vi "SyringeZCalibration.vi"(4 "AssmbType":enum16{"Sensor", "HB"}(ring), 5 "ModuleName":string="T1", 6 "Position":enum16{"1", "2"}(ring), 7 "Zone":enum16{"ZoneA", "ZoneB", "ZoneC", "ZoneD"}(ring), 8 "Error In":errorcluster, 9 "SyringeToPlateGap(mm)":dbl=0.35, 10 "PD_Z":bool=TRUE, 11 "AutoFocus":bool=TRUE) -> (0 "error out":errorcluster, 1 "HighVSPosition":picture, 2 "Image":T2(plugin-control), 3 "FinalZ":dbl)   [LabVIEW 2019]
uses:
  <vilib>/Utility/file.llb/Read Delimited Spreadsheet (DBL).vi
  include/GlobalVariables.vi
panel:
  out "CurrentZvalue":dbl
  out "AF_Zs":string
  out "SyringeZwriteTo":string
  out "OffsetUsed":dbl
  in  "Offset = -(AF_Z + PD_Z - FinalZ_needed - Gap)":T1={"BP_Zoffset(Si_assembly)"=-68.2905, "Sensor_Zoffset(HB_assembly)"=-68.3505}
  out "AF_MinZ":dbl
  out "AF_OutputPlotFile":string
  out "AF_OutputTextFile":string
  out "AF_InputTextFile":string
  out "VatPD_Z":dbl
  out "MeasuredPD_Z":dbl
  out "Vmid":dbl
  out "Vmin":dbl
  out "Vstart":dbl
  out "Vmax":dbl
  # "MainInputs"
  # "MainOutputs"
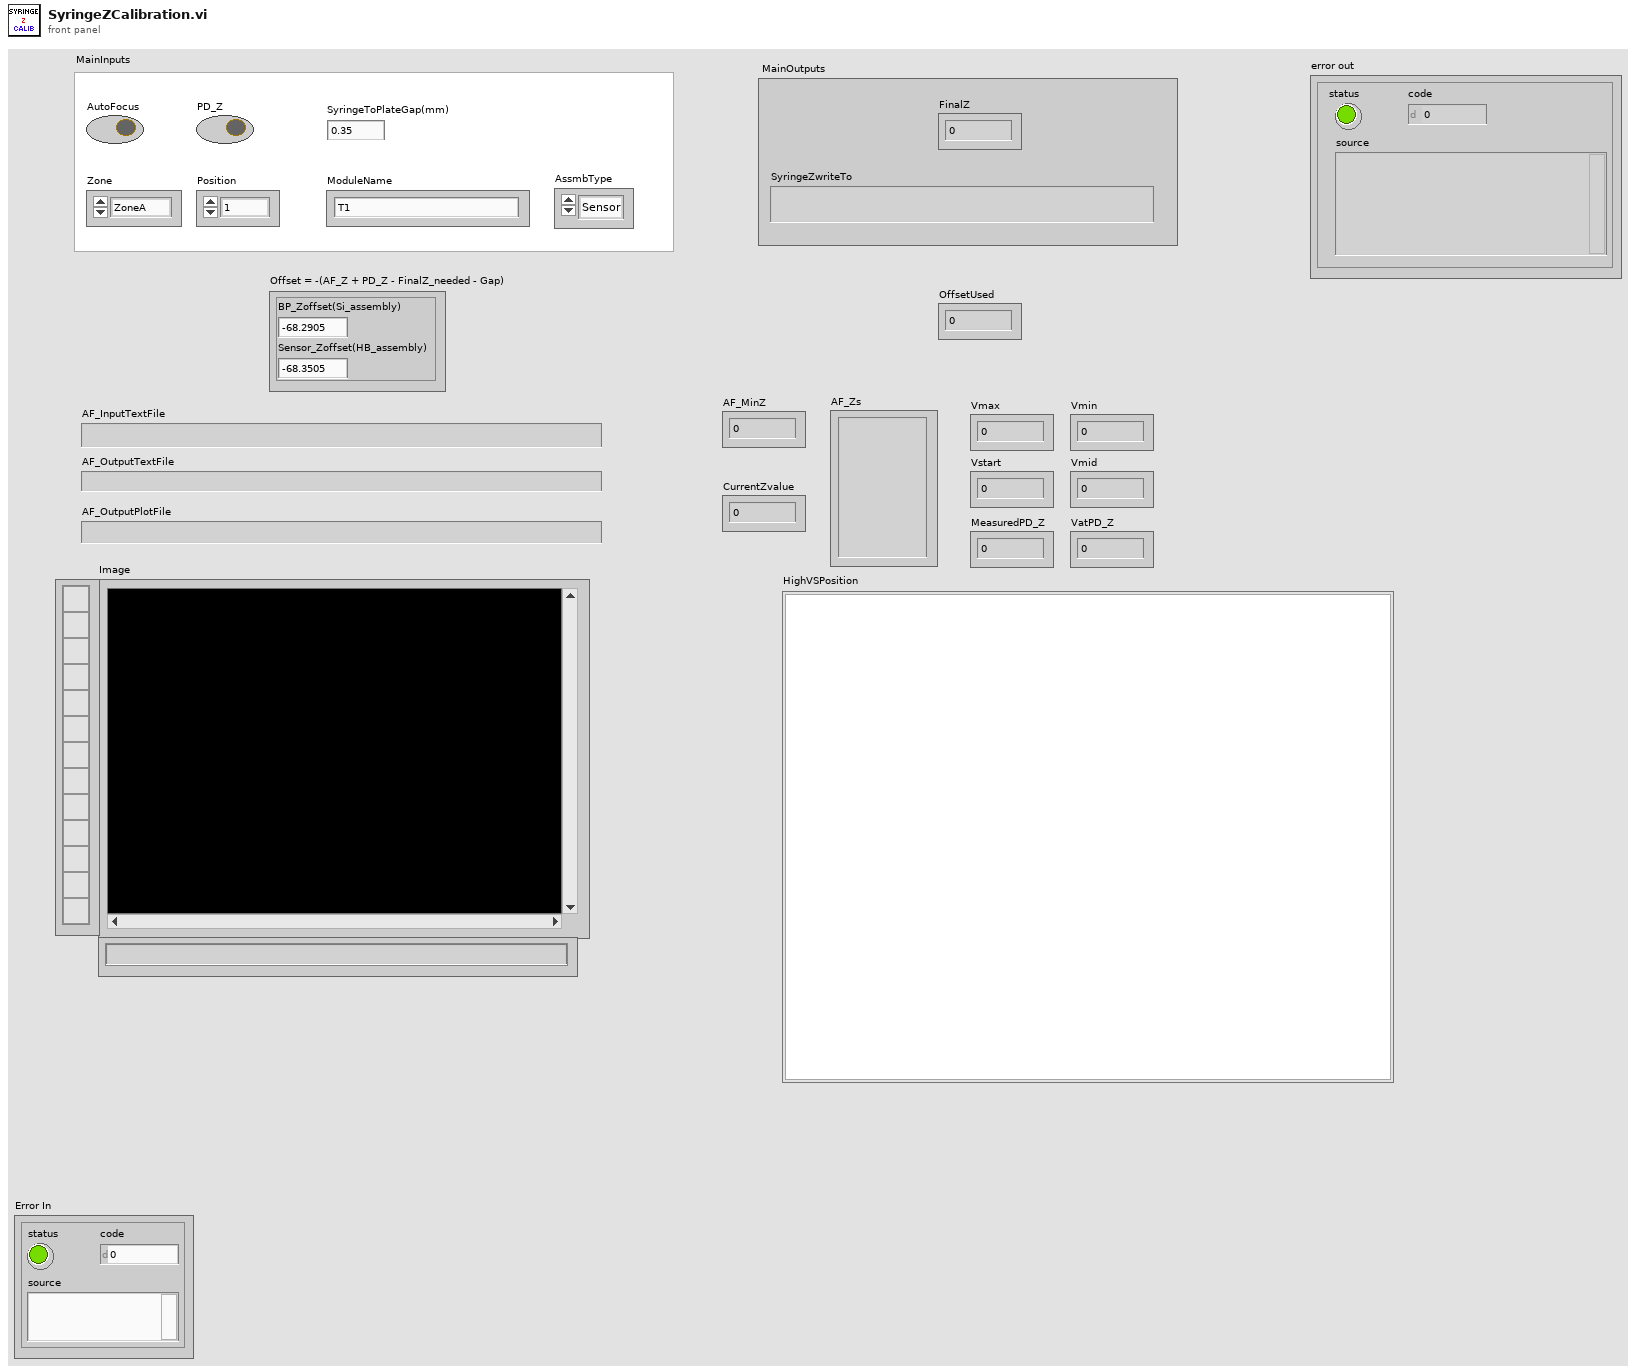
[diagram p1: front panel]
types:
  T1 = cluster{"BP_Zoffset(Si_assembly)":dbl, "Sensor_Zoffset(HB_assembly)":dbl}
  T2 = typedef "IMAQ Image.ctl" = refnum<image>
  T3 = enum16{"open", "replace", "create", "open or create", "replace or create", "replace or create with confirmation"}
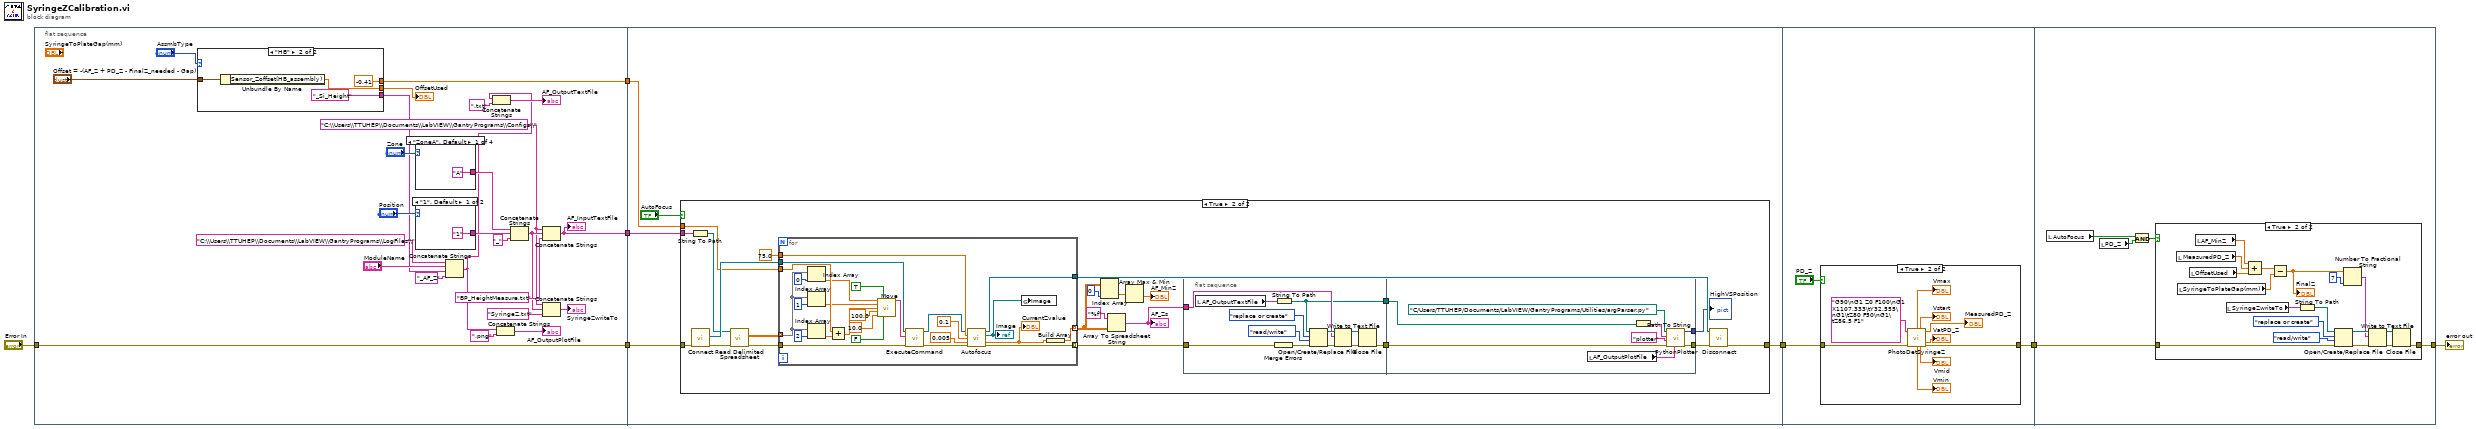
[diagram p0: block diagram]
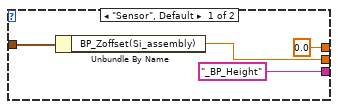
[diagram p2: hidden frame]
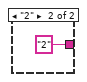
[diagram p3: hidden frame]
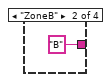
[diagram p4: hidden frame]
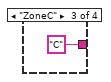
[diagram p5: hidden frame]
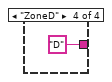
[diagram p6: hidden frame]
diagram:
  n1 = flat-sequence {
    tunnel: "Error In" -> [w20]
    tunnel: [w20] -> w5
    tunnel: [w27] -> w4
    tunnel: [w25] -> w3
    tunnel: w5 -> [w51]
    tunnel: w4 -> [w48]
    tunnel: w3 -> [w47]
    tunnel: [w49] -> w2
    tunnel: w2 -> [w122]
    tunnel: [w121] -> w1
    tunnel: [w134] -> w7
    tunnel: w1 -> [w135]
    frame #0 {
      w12 = "C:\\Users\\TTUHEP\\Documents\\LabVIEW\\GantryPrograms\\Configs\\"
      n2 = case shown="\"HB\"" "AssmbType" {
        tunnel: [0.0 -0.41] -> w27
        tunnel: "Offset = -(AF_Z + PD_Z - FinalZ_needed - Gap)" -> [w35 w39]
        tunnel: [w34 w38] -> w9
        tunnel: ["_BP_Height" "_Si_Height"] -> w8
        frame "Sensor", Default {
          n3 = Unbundle By Name(w35) -> ("BP_Zoffset(Si_assembly)"=w34:dbl)
        }
        frame "HB" {
          n4 = Unbundle By Name(w39) -> ("Sensor_Zoffset(HB_assembly)"=w38:dbl)
        }
      }
      "OffsetUsed" <- w9
      n5 = case shown="\"ZoneA\", Default" "Zone" {
        tunnel: ["A" "B" "C" "D"] -> w31
        frame "ZoneA", Default {
        }
        frame "ZoneB" {
        }
        frame "ZoneC" {
        }
        frame "ZoneD" {
        }
      }
      n6 = case shown="\"1\", Default" "Position" {
        tunnel: ["1" "2"] -> w32
        frame "1", Default {
        }
        frame "2" {
        }
      }
      n7 = Concatenate Strings("C:\\Users\\TTUHEP\\Documents\\LabVIEW\\GantryPrograms\\LogFiles\\", "ModuleName", w8, "_AF_Z" ("string")) -> (w16:string)
      n8 = Concatenate Strings(w16, ".txt" ("string")) -> (→"AF_OutputTextFile":string)
      n9 = Concatenate Strings(w16, ".png" ("string")) -> (→"AF_OutputPlotFile":string)
      n10 = Concatenate Strings(w31, w32, "_" ("string")) -> (w14:string)
      n11 = Concatenate Strings(w12, w14, "BP_HeightMeasure.txt" ("string")) -> (w25:string)
      "AF_InputTextFile" <- w25
      n12 = Concatenate Strings(w12, w14, "SyringeZ.txt" ("string")) -> (→"SyringeZwriteTo":string)
    }
    frame #1 {
      n13 = case shown="True" "AutoFocus" {
        tunnel: w51 -> [w52 w61]
        tunnel: [w52 w60] -> w49
        tunnel: w48 -> [_ w59]
        tunnel: w47 -> [_ w57]
        frame False {
        }
        frame True {
          n14 = String To Path(string=w57) -> (path=w58:path)
          n15 = call "Connect.vi"("error in (no error)"=w61) -> ("error out"=w71:errorcluster, "controller"=w72:refnum<k24>)  [unwired: 9 in]
          n16 = call-poly <vilib>:"Read Delimited Spreadsheet.vi"("file path (dialog if empty)"=w58, "error in (no error)"=w71) -> ("all rows"=w67:dbl[][], "error out"=w63:errorcluster)  [unwired: 8 in, 4 out]
          n17 = for {
            tunnel: w67 -> [w117] mode=indexing
            tunnel: w63 -> [w99]
            tunnel: [w115] -> w66 mode=indexing
            tunnel: [w114] -> w55 mode=indexing
            tunnel: w72 -> [w101]
            tunnel: [w113] -> w69
            tunnel: 75.0 ("SafeMaxZ") -> [w110]
            tunnel: w59 -> [w112]
            n18 = Index Array(array=w117, index=0) -> (element=w109:dbl)
            n19 = Index Array(array=w117, index=1) -> (element=w108:dbl)
            n20 = Index Array(array=w117, index=2) -> (element=w111:dbl)
            n21 = Add(x=w112, y=w111) -> (x+y=w107:dbl)
            n22 = call "Move.vi"("X"=w109, "Absolute"=TRUE, "Y"=w108, "Z"=w107, "SpeedXY (mm/s)"=100.0, "SpeedZ (mm/s)"=10.0, "Move Z first"=FALSE) -> ("Position Gcode"=w102:string)  [unwired: 8 in]
            n23 = call "ExecuteCommand.vi"("error in (no error)"=w99, "Command Code"=w102, "controller in"=w101) -> ("error out"=w98:errorcluster, "controller out"=w100:refnum<k24>)  [unwired: 6 in, 1 out]
            n24 = call "Autofocus.vi"("controller in"=w100, "SafeMaxZ"=w110, "InitialStepSize"=0.1, "Tolerance"=0.005, "error in (no error)"=w98) -> ("controller out"=w113:refnum<k24>, "Image"=w95:T2, "BestZvalue"=w116:dbl, "error out"=w115:errorcluster)  [unwired: 6 in, 1 out]
            "Image" <- w95
            "CurrentZvalue" <- w116
            n25 = global write "GlobalVariables.vi" "Image"(w95) -> ()
            n26 = Build Array(w116) -> (w114:dbl[])
          }
          n27 = Index Array(array=w55, index (col)=0 ("disabled index (col)")) -> (element=w53:dbl[])  [unwired: 1 in]
          n28 = Array To Spreadsheet String(array=w55, 3:"%f" ("format string")) -> (spreadsheet string=w64:string)  [unwired: 1 in]
          "AF_Zs" <- w64
          n29 = Array Max & Min(array=w53) -> (min value=→"AF_MinZ":dbl)  [unwired: 3 out]
          n30 = flat-sequence {
            tunnel: w66 -> [w86]
            tunnel: w64 -> [w79]
            tunnel: [w77] -> w74
            tunnel: [w76] -> w73
            tunnel: w74 -> [w94]
            tunnel: [w93] -> w70
            tunnel: [w92] -> w62
            tunnel: w73 -> [w89]
            frame #0 {
              n31 = local read "AF_OutputTextFile"() -> (w75:string)
              n32 = Merge Errors(w86) -> (w78:errorcluster)
              n33 = String To Path(string=w75) -> (path=w76:path)
              n34 = Open/Create/Replace File(file path (use dialog)=w76, error in=w78, operation (0:open)=T3."replace or create", access (0:read/write)=enum16{"read/write", "read-only", "write-only"}."read/write") -> (refnum out=w82:refnum<file>, error out=w83:errorcluster)  [unwired: 2 in, 1 out]
              n35 = Write to Text File(file (use dialog)=w82, text=w79, error in=w83) -> (refnum out=w85:refnum<file>, error out=w84:errorcluster)  [unwired: 1 in, 1 out]
              n36 = Close File(refnum=w85, error in=w84) -> (error out=w77:errorcluster)  [unwired: 1 out]
            }
            frame #1 {
              n37 = local read "AF_OutputPlotFile"() -> (w87:string)
              n38 = Path To String(path=w89) -> (string=w90:string)
              n39 = call "PythonPlotter.vi"("Output File"=w87, "error in (no error)"=w94, "Function Name"="plotter", "Input File"=w90, "Python Path"=path "C:/Users/TTUHEP/Documents/LabVIEW/GantryPrograms/Utilities/argParser.py") -> ("error out"=w93:errorcluster, "HighVSPosition"=w92:picture)  [unwired: 4 in]
            }
          }
          n40 = call "Disconnect.vi"("error in (no error)"=w70, "controller"=w69) -> ("error out"=w60:errorcluster)  [unwired: 9 in]
          "HighVSPosition" <- w62
        }
      }
    }
    frame #2 {
      n41 = case shown="True" "PD_Z" {
        tunnel: [w124 w126] -> w121
        tunnel: w122 -> [w124 w125]
        frame False {
        }
        frame True {
          n42 = call "PhotoDetSyringeZ.vi"("GoToPhotoDetector"="G90\nG1 Z0 F100\nG1 X1107.333\tY32.555\nG1\tZ80 F50\nG1\tZ86.5 F1", "Error In"=w125) -> ("Vmax"=→"Vmax":dbl, "Vstart"=→"Vstart":dbl, "Zfinal"=→"MeasuredPD_Z":dbl, "VatZfinal"=→"VatPD_Z":dbl, "Vmin"=→"Vmin":dbl, "Vmid"=→"Vmid":dbl, "error out"=w126:errorcluster)  [unwired: 7 in]
        }
      }
    }
    frame #3 {
      n43 = local read "AutoFocus"() -> (w138:bool)
      n44 = local read "PD_Z"() -> (w137:bool)
      n45 = And(x=w138, y=w137) -> (x .and. y?=w136:bool)
      n46 = case shown="True" w136 {
        tunnel: w135 -> [w139 w141]
        tunnel: [w139 w140] -> w134
        frame False {
        }
        frame True {
          n47 = local read "MeasuredPD_Z"() -> (w156:dbl)
          n48 = local read "SyringeToPlateGap(mm)"() -> (w153:dbl)
          n49 = local read "OffsetUsed"() -> (w155:dbl)
          n50 = local read "AF_MinZ"() -> (w157:dbl)
          n51 = local read "SyringeZwriteTo"() -> (w146:string)
          n52 = Compound Arithmetic op=ADD(w157, w156, w155) -> (w154:dbl)
          n53 = Subtract(x=w154, y=w153) -> (x-y=w144:dbl)
          "FinalZ" <- w144
          n54 = String To Path(string=w146) -> (path=w145:path)
          n55 = Open/Create/Replace File(file path (use dialog)=w145, error in=w141, operation (0:open)=T3."replace or create", access (0:read/write)=enum16{"read/write", "read-only", "write-only"}."read/write") -> (refnum out=w152:refnum<file>, error out=w149:errorcluster)  [unwired: 2 in, 1 out]
          n56 = Number To Fractional String(number=w144, precision (6)=i16 7) -> (F-format string=w142:string)  [unwired: 2 in]
          n57 = Write to Text File(file (use dialog)=w152, text=w142, error in=w149) -> (refnum out=w147:refnum<file>, error out=w148:errorcluster)  [unwired: 1 in, 1 out]
          n58 = Close File(refnum=w147, error in=w148) -> (error out=w140:errorcluster)  [unwired: 1 out]
        }
      }
    }
  }
  "error out" <- w7
